vi "Set End Time.vi"(8 "error in (no error)":errorcluster, 10 "End Time":timestamp, 11 "Test Result in":refnum<class "Test Result.lvclass">) -> (0 "error out":errorcluster, 3 "Test Result out":refnum<class "Test Result.lvclass">)   [LabVIEW 2017, in "Test Result.lvclass"]
uses:
  Test Result.lvclass
  Test Result.lvclass/Test Result.ctl
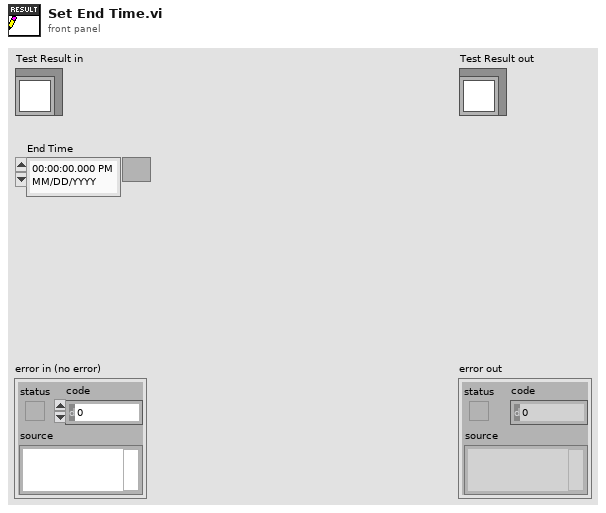
[diagram p1: front panel]
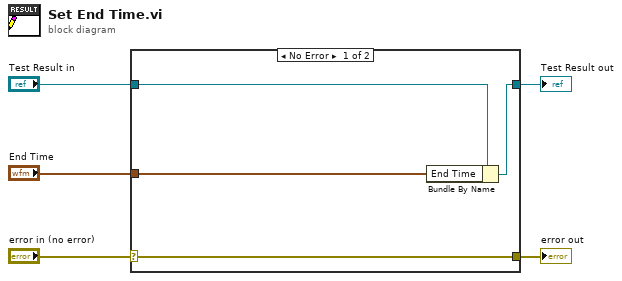
[diagram p0: block diagram]
diagram:
  n1 = case shown="No Error" "error in (no error)" {
    selector: "error in (no error)" -> [w9 w10]
    tunnel: [w9 w10] -> w4
    tunnel: [w7 w11] -> w2
    tunnel: "Test Result in" -> [w8 w11]
    tunnel: "End Time" -> [w6 _]
    frame No Error {
      n2 = Bundle By Name(cluster=w8, "End Time"=w6) -> (w7:refnum<class "Test Result.lvclass">)
    }
    frame Error {
    }
  }
  "error out" <- w4
  "Test Result out" <- w2
